vi "Test Timed Door API.vi"() -> ()   [LabVIEW 2018]
uses:
  Timed Door.lvclass
  Set Target Time (seconds).vi
panel:
  out "error out":errorcluster
  in  "Timed Door Target Time (seconds)":dbl=5.0
  in  "Door Switch":enum32{"Open Door", "Close Door"}(radio)=enum."Close Door"
  out "Door":u16(ring)
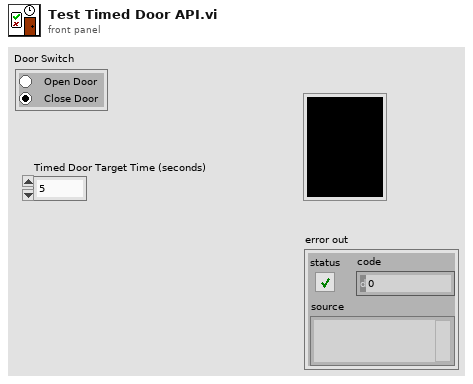
[diagram p1: front panel]
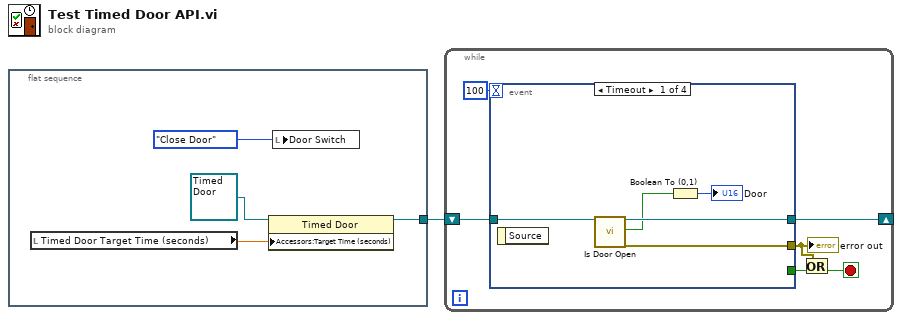
[diagram p0: block diagram]
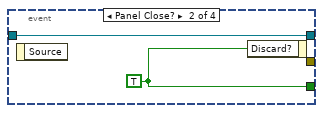
[diagram p2: hidden frame]
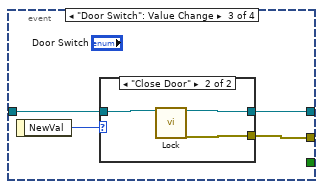
[diagram p3: hidden frame]
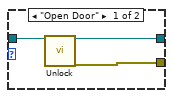
[diagram p4: hidden frame]
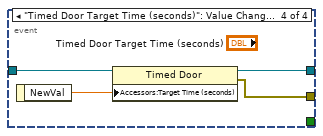
[diagram p5: hidden frame]
diagram:
  n1 = flat-sequence {
    tunnel: [w3] -> w1
    frame #0 {
      n2 = local read "Timed Door Target Time (seconds)"() -> (w4:dbl)
      n3 = property class="Timed Door"(reference=refnum<class "Timed Door.lvclass"> refnum ("Timed Door.lvclass"), "Accessors:Target Time (seconds)"=w4) -> (reference out=w3:refnum<class "Timed Door.lvclass">)  [unwired: 1 in, 1 out]
      n4 = local write "Door Switch"(enum32{"Open Door", "Close Door"}."Close Door" ("Door Switch")) -> ()
    }
  }
  n5 = while {
    shift-right: [w8] -> _
    shift-left: w1 -> [w10]
    stop <- w7 stop-if-true
    n6 = event shown="[0] Timeout" {
      selector: _ -> [_ _ _ _]
      dyn-events: _ -> [_ _ _ _]
      timeout: 100 -> [_ _ _ _]
      tunnel: w10 -> [w15 w17 w22 w30]
      tunnel: [_ w18 _ _] -> w9
      tunnel: [w14 w17 w21 w32] -> w8
      tunnel: [w12 _ w19 w29] -> w6
      event Timeout {
        n7 = event-data() -> ()  [unwired: 1 in, 1 out]
        n8 = call-dynamic "Is Door Open.vi"("Interface_object in"=w15) -> ("Interface_object out"=w14:refnum<class "Timed Door.lvclass">, "Is Door Open?"=w13:bool, "error out"=w12:errorcluster)  [unwired: 16 in]
        n9 = Boolean To (0,1)(Boolean=w13) -> (0, 1=→"Door":i16)
      }
      event Panel Close? {
        w18 = TRUE ("Discard?")
        n10 = event-data() -> ()  [unwired: 1 in, 1 out]
        n11 = event-data("Discard?"=w18) -> ()  [unwired: 1 in, 1 out]
      }
      event "Door Switch": Value Change {
        n12 = event-data() -> ("NewVal"=w20:enum32{"Open Door", "Close Door"})  [unwired: 1 in]
        n13 = case shown="\"Close Door\"" w20 {
          tunnel: w22 -> [w25 w28]
          tunnel: [w24 w27] -> w21
          tunnel: [w23 w26] -> w19
          frame "Open Door" {
            n14 = call-dynamic "Unlock.vi"("Interface_object in"=w25) -> ("Interface_object out"=w24:refnum<class "Timed Door.lvclass">, "error out"=w23:errorcluster)  [unwired: 17 in]
          }
          frame "Close Door" {
            n15 = call-dynamic "Lock.vi"("Interface_object in"=w28) -> ("Interface_object out"=w27:refnum<class "Timed Door.lvclass">, "error out"=w26:errorcluster)  [unwired: 17 in]
          }
        }
      }
      event "Timed Door Target Time (seconds)": Value Change {
        n16 = event-data() -> ("NewVal"=w31:dbl)  [unwired: 1 in]
        n17 = property class="Timed Door"(reference=w30, "Accessors:Target Time (seconds)"=w31) -> (reference out=w32:refnum<class "Timed Door.lvclass">, error out=w29:errorcluster)  [unwired: 1 in]
      }
    }
    "error out" <- w6
    n18 = Or(x=w6, y=w9) -> (x .or. y?=w7:bool)
  }
